vi "AlliGator Fit Linear Combinations of Exponentials.vi"(0 "Simulation Parameters":T1={"Decay Simulation Parameters"={"tau 1"=1e-09, "tau 2"=0.0, "a1"=1.0, "Baseline"=0.0}, "Fit Simulation Parameters"={"# Counts"=100, "# Simulations (N)"=100, "Decay Bin Size"=1.0000000000000002e-10, "# Bins"=200}, "Use Experimental IRF"=FALSE}, 5 "Decay Fit Options & Parameters":T5={"SYNC Period"=0.0, "Fit Options"={"Show Fit Residuals"=FALSE, "Fit Model"=enum."1-Exponential", "Residual Type"=enum."Standard", "Max Decay Percentile"=0.0, "Min Decay Percentile"=0.0, "Show Full Decay"=FALSE, "Weights"=enum."Unweighted", "Fitting Method"=enum."Least Square", "Compute Parameter Uncertainties"=FALSE, "Periodic Boundaries"=FALSE, "Model Calculation"=enum."Simulation", "Period"=0.0, "Termination Criteria"={"Max Iterations"=0, "Max Function Calls"=0, "Max Time"=0.0, "Function Tolerance"=0.0, "Parameter Tolerance"=0.0, "Gradient Tolerance"=0.0, "Min Lambda"=0.0, "Max Lambda"=0.0, "Initial Tick Count"=0}, "Offset Resolution"=0.0, "Use Local IRF"=FALSE, "Fitting Algorithm"=enum."Levenberg-Marquardt", "Show Confidence Interval "=TRUE, "Confidence Level"=95.0}, "Fit Parameter Constraints"=[], "MLE Baseline Offset"=0.0, "MLE Baseline Offset Type"=enum."Absolute"} {"Fit Options"."Confidence Level" min=0.0 max=100.0; "Fit Options"."Offset Resolution" min=0.0; "Fit Options"."Period" min=0.0; "Fit Options"."Min Decay Percentile" min=0.0 max=1.0; "Fit Options"."Max Decay Percentile" min=0.0 max=100.0; "Fit Parameter Constraints"."Max Value" format="%#.3g"; "Fit Parameter Constraints"."Min Value" format="%#.3g"}, 9 "Reference Decay":cluster{"t Array":dbl[], "IRF Array":dbl[]}, 11 "Error In":errorcluster, 12 "Show Decays, Fits & Residuals":bool) -> (1 "Output Plots":cluster{"t Array":dbl[], "I Array":dbl[]}[](array[cluster]), 2 "Output Plot Names":string[](array[string]), 3 "Plot Colors":u32[](array[colorbox]), 4 "Fit Results":T4[](array[typedef]), 6 "tau 1":dbl[](array[numeric]), 8 "tau 2":dbl[](array[numeric]), 10 "a 1":dbl[](array[numeric]), 14 "Message":string, 15 "Error Out":errorcluster)   [LabVIEW 2021, in "AlliGator Fit Method Benchmark.lvlib"]
doc: "Simulate a 1-Exp or 2-Exp decay and fits it with the selected model."
uses:
  AlliGator Fit Method Benchmark.lvlib
  Histograms/Histogram Bin Option.ctl
  Histograms/Histogram Window.lvlib
  Histograms/Histogram Bin Position.ctl
  Histograms/Linear Histogram Options.ctl
  Math/Math.lvlib
  GUI/GUI.lvlib
  Globals, Variables, Constants/AlliGator Abort.vi
  Globals, Variables, Constants/AlliGator Globals, Variables & Constants.lvlib
  Time/Time.lvlib
  Variant/Variant.lvlib
  Decay Analysis/Decay Fit/AlliGator Decay Fit.lvlib
  Graphs/XY Graph/XY Graph Refnum.ctl
  Graphs/XY Graph/XY Graph Add-Ons.lvlib
  <vilib>/Utility/miscctls.llb/LVPoint32TypeDef.ctl
  Graphs/XY Graph/XY Graph Selected Plot Info+Flag.ctl
  Fits/IRF(X)PSED/IRF(X)PSED Fit Results.ctl
  Fits/Fits.lvlib
  <vilib>/gmath/NI_Gmath.lvlib
  <vilib>/ErrorRing/Error Ring.xnode
  <vilib>/Utility/error.llb/Error Cluster From Error Code.vi
  Error/Error.lvlib
  <vilib>/gmath/statdist.llb/Exp Random.vi
  <vilib>/gmath/statdist.llb/Uniform (Discrete) Random.vi
  593261b4-01b2-4f61-a03e-748a91d26851.vi
  AlliGator FMB Global.vi
  AlliGator Fit Simulation Parameters.ctl
  AlliGator Decay Simulation Parameters.ctl
  Fits/IRF(X)PSED/Decay Fit Parameters In List.ctl
  Decay Analysis/Decay Fit/AlliGator Decay Fit Parameter Constraints 2.ctl
  Fits/Decay Convolution/Decay Model.ctl
  Fits/Residual Type.ctl
  Fits/Non-linear Fitting Method v2.ctl
  Fits/Fit Calculation Method.ctl
  Fits/Non-linear Fitting Algorithm.ctl
  Fits/IRF(X)PSED/MLE Baseline Offset Type.ctl
  AlliGator Simulation Parameters.ctl
  Fits/IRF(X)PSED/Fit Weights Type v2.ctl
  Fits/IRF(X)PSED/Decay Fit Options v4.ctl
  Decay Fit Parameter Map/AlliGator Decay Fit Options & Parameters v4.ctl
  Decay Fit Parameter Map/AlliGator Decay Fit Parameter Map.lvlib
panel:
  # "see the AlliGator License on the block diagram (Ctrl+E or Window:Show Block Diagram)"
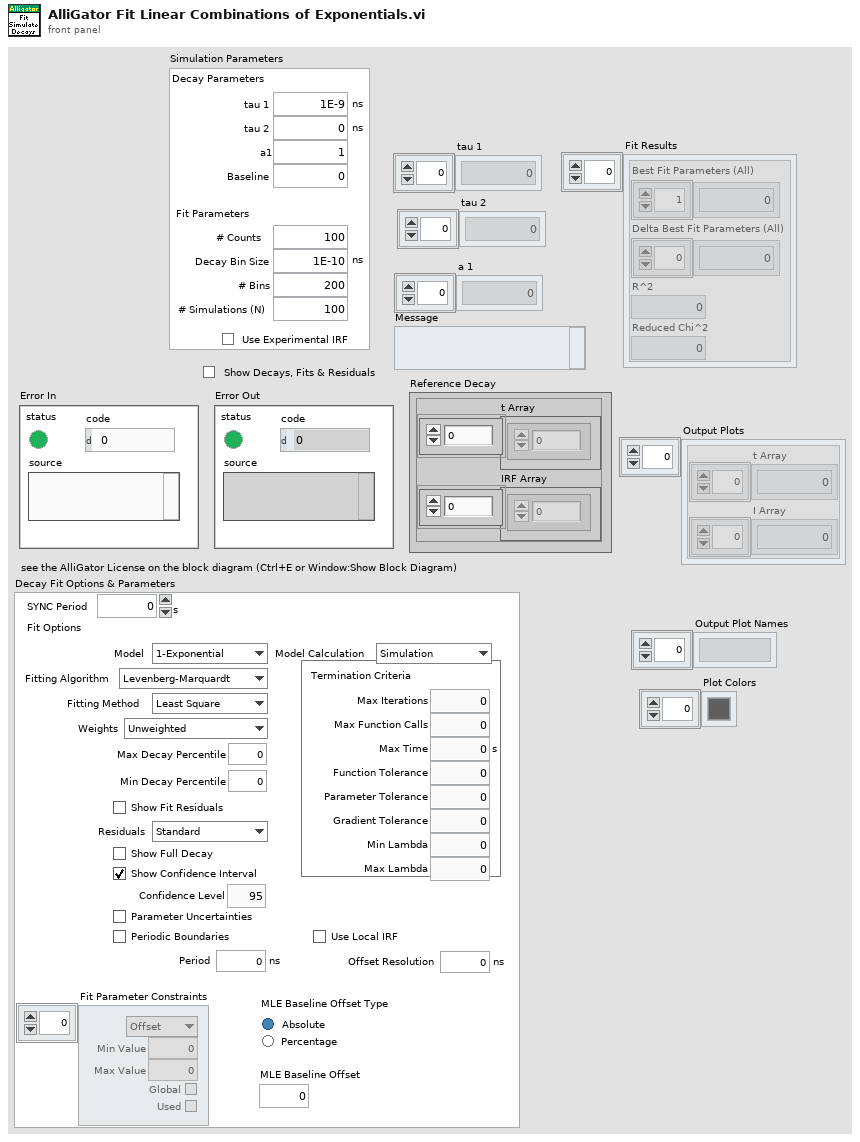
[diagram p1: front panel]
types:
  T1 = typedef "AlliGator Fit Method Benchmark.lvlib/AlliGator Simulation Parameters.ctl" = cluster{"Decay Simulation Parameters":T2, "Fit Simulation Parameters":T3, "Use Experimental IRF":bool}
  T2 = typedef "AlliGator Fit Method Benchmark.lvlib/AlliGator Decay Simulation Parameters.ctl" = cluster{"tau 1":dbl[unit], "tau 2":dbl[unit], "a1":dbl, "Baseline":dbl}
  T3 = typedef "AlliGator Fit Method Benchmark.lvlib/AlliGator Fit Simulation Parameters.ctl" = cluster{"# Counts":i32, "# Simulations (N)":i32, "Decay Bin Size":dbl[unit], "# Bins":i32}
  T4 = typedef "Fits.lvlib/IRF(X)PSED Fit Results.ctl" = cluster{"Best Fit Parameters (All)":dbl[], "Delta Best Fit Parameters (All)":dbl[], "R^2":dbl, "Reduced Chi^2":dbl}
  T5 = typedef "AlliGator Decay Fit Parameter Map.lvlib/AlliGator Decay Fit Options & Parameters v4.ctl" = cluster{"SYNC Period":dbl[unit], "Fit Options":T6, "Fit Parameter Constraints":T13[], "MLE Baseline Offset":dbl, "MLE Baseline Offset Type":T15}
  T6 = typedef "Fits.lvlib/Decay Fit Options v4.ctl" = cluster{"Show Fit Residuals":bool, "Fit Model":T7, "Residual Type":T8, "Max Decay Percentile":dbl, "Min Decay Percentile":dbl, "Show Full Decay":bool, "Weights":T9, "Fitting Method":T10, "Compute Parameter Uncertainties":bool, "Periodic Boundaries":bool, "Model Calculation":T11, "Period":dbl[unit], "Termination Criteria":cluster{"Max Iterations":i32, "Max Function Calls":i32, "Max Time":dbl[unit], "Function Tolerance":dbl, "Parameter Tolerance":dbl, "Gradient Tolerance":dbl, "Min Lambda":dbl, "Max Lambda":dbl, "Initial Tick Count":u32}, "Offset Resolution":dbl[unit], "Use Local IRF":bool, "Fitting Algorithm":T12, "Show Confidence Interval ":bool, "Confidence Level":dbl}
  T7 = typedef "Fits.lvlib/Decay Model.ctl" = enum16{"1-Exponential", "2-Exponentials"}
  T8 = typedef "Fits.lvlib/Residual Type.ctl" = enum16{"Standard", "Normalized", "Reduced"}
  T9 = typedef "Fits.lvlib/Fit Weights Type v2.ctl" = enum16{"Unweighted", "1/Variance (Neyman)", "1/Variance (Pearson)", "Best of All"}
  T10 = typedef "Fits.lvlib/Non-linear Fitting Method v2.ctl" = enum16{"Least Square", "Least Absolute Residual", "Bisquare", "MLE", "-", "Best of All"}
  T11 = typedef "Fits.lvlib/Fit Calculation Method.ctl" = enum16{"Simulation", "Convolution", "Integration"}
  T12 = typedef "Fits.lvlib/Non-linear Fitting Algorithm.ctl" = enum16{"Levenberg-Marquardt", "Trust-Region Dogleg"}
  T13 = typedef "AlliGator Decay Fit.lvlib/AlliGator Decay Fit Parameter Constraints 2.ctl" = cluster{"Fit Parameter":T14, "Min Value":dbl, "Max Value":dbl, "Global":bool, "Used":bool}
  T14 = typedef "Fits.lvlib/Decay Fit Parameters In List.ctl" = enum16{"Offset", "Baseline", "A_1", "tau_1", "A_2", "tau_2"}
  T15 = typedef "Fits.lvlib/MLE Baseline Offset Type.ctl" = enum32{"Absolute", "Percentage"}
  T16 = typedef "Histogram Window.lvlib/Linear Histogram Options.ctl" = cluster{"Bin Size":dbl, "Bin Number":i32, "Bin Option":T17, "Min Value":dbl, "Max Value":dbl, "Filter NaN & Infinite Values":bool, "Frequency Plot":bool, "Align Bins":bool, "Bin Location":T18, "Project Outside Values":bool, "Max Histogram Size":i32}
  T17 = typedef "Histogram Window.lvlib/Histogram Bin Option.ctl" = enum32{"Bin Number", "Bin Size"}
  T18 = typedef "Histogram Window.lvlib/Histogram Bin Position.ctl" = enum16{"Left", "Center", "Right"}
  T19 = typedef "XY Graph Add-Ons.lvlib/XY Graph Selected Plot Info+Flag.ctl" = cluster{"Multiplot XY Graph":T20, "Mouse Coordinates":T21, "Plot Index":i32, "Flag":bool}
  T20 = typedef "XY Graph Add-Ons.lvlib/XY Graph Refnum.ctl" = refnum<vi>
  T21 = typedef "LVPoint32TypeDef.ctl" = cluster{"Horizontal":i32, "Vertical":i32}
  T22 = typedef "XY Graph Add-Ons.lvlib/XY Graph Plot Data.ctl" = cluster{"X Array":dbl[], "Y Array":dbl[]}
  T23 = typedef "Fits.lvlib/Fit Plots.ctl" = cluster{"Fitted Decay":cluster{"t Array":dbl[], "Fitted Array":dbl[]}, "Residuals":cluster{"t Array":dbl[], "Residual Array":dbl[]}, "Upper CI Plot":cluster{"t Array":dbl[], "Residual Array":dbl[]}, "Lower CI Plot":cluster{"t Array":dbl[], "Residual Array":dbl[]}}
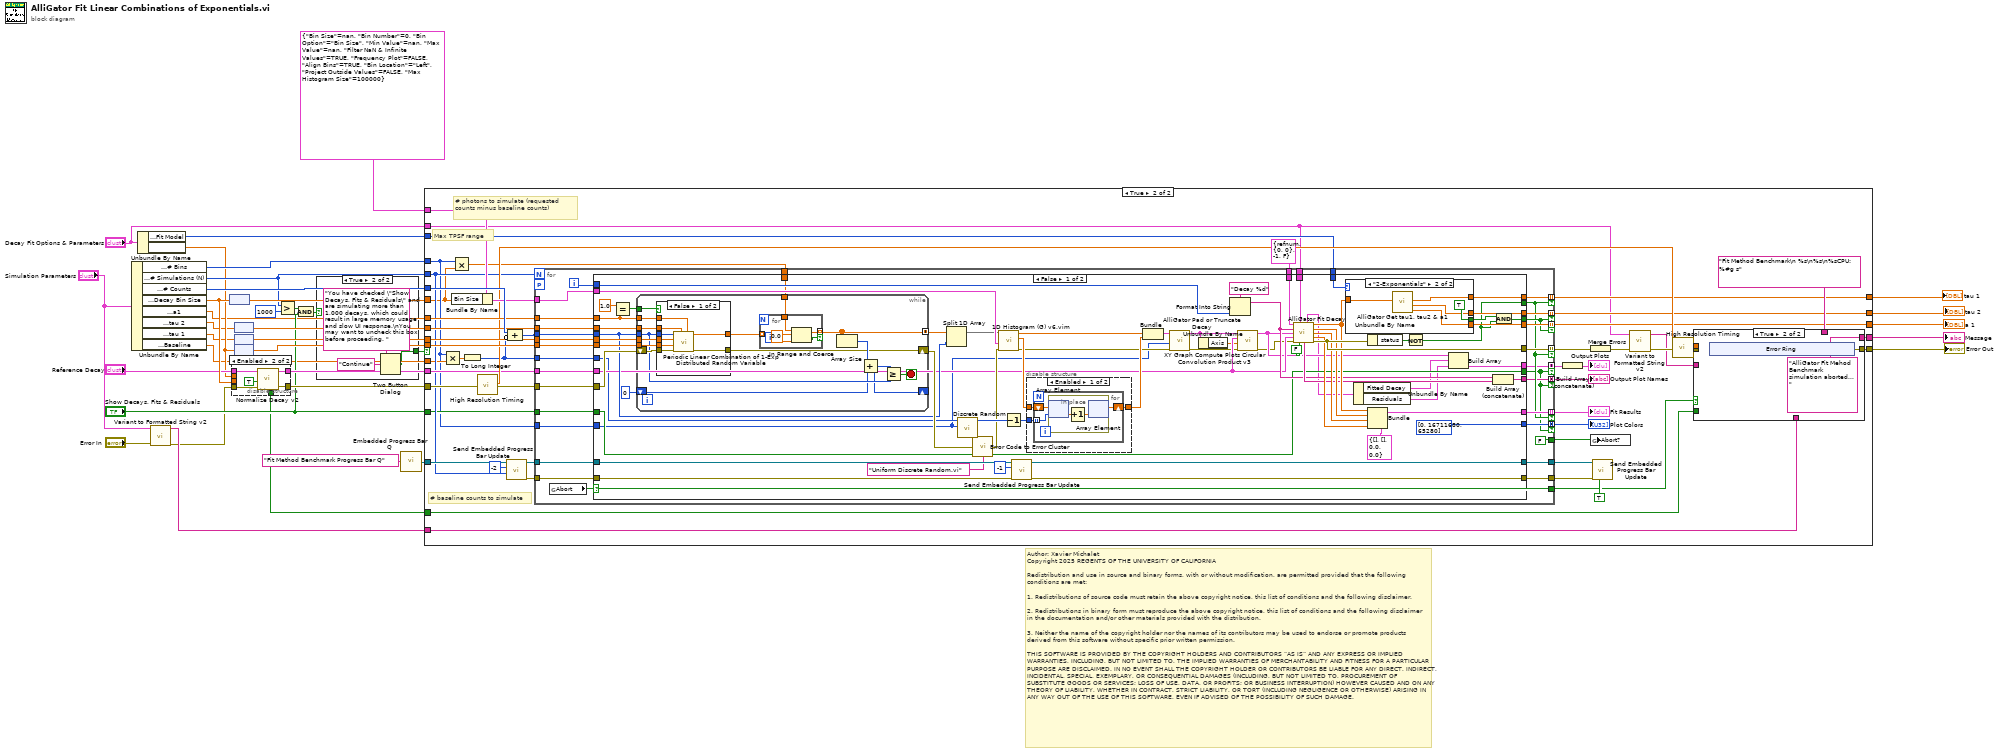
[diagram p0: block diagram]
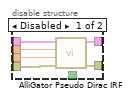
[diagram p2: hidden frame]
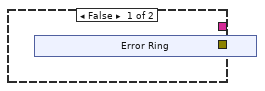
[diagram p3: hidden frame]
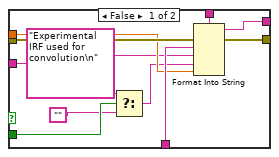
[diagram p4: hidden frame]
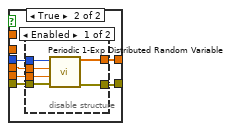
[diagram p5: hidden frame]
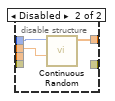
[diagram p6: hidden frame]
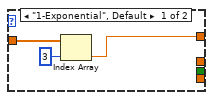
[diagram p8: hidden frame]
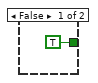
[diagram p10: hidden frame]
diagram:
  # "Author: Xavier Michalet\nCopyright 2025 REGENTS OF THE UNIVERSITY OF CALIFORNIA\n\nRedistribution and use in source and binary forms, with or without modification, are permitted provided that the following conditions are met:\n\n1. Redistributions of source code must retain the above copyright notice, this list of conditions and the following disclaimer.\n\n2. Redistributions in binary form must reproduce the above copyright notice, this list of conditions and the following disclaimer in the documentation and/or other materials provided with the distribution.\n\n3. Neither the name of the copyright holder nor the names of its contributors may be used to endorse or promote products derived from this software without specific prior written permission.\n\nTHIS SOFTWARE IS PROVIDED BY THE COPYRIGHT HOLDERS AND CONTRIBUTORS “AS IS” AND ANY EXPRESS OR IMPLIED WARRANTIES, INCLUDING, BUT NOT LIMITED TO, THE IMPLIED WARRANTIES OF MERCHANTABILITY AND FITNESS FOR A PARTICULAR PURPOSE ARE DISCLAIMED. IN NO EVENT SHALL THE COPYRIGHT HOLDER OR CONTRIBUTORS BE LIABLE FOR ANY DIRECT, INDIRECT, INCIDENTAL, SPECIAL, EXEMPLARY, OR CONSEQUENTIAL DAMAGES (INCLUDING, BUT NOT LIMITED TO, PROCUREMENT OF SUBSTITUTE GOODS OR SERVICES; LOSS OF USE, DATA, OR PROFITS; OR BUSINESS INTERRUPTION) HOWEVER CAUSED AND ON ANY THEORY OF LIABILITY, WHETHER IN CONTRACT, STRICT LIABILITY, OR TORT (INCLUDING NEGLIGENCE OR OTHERWISE) ARISING IN ANY WAY OUT OF THE USE OF THIS SOFTWARE, EVEN IF ADVISED OF THE POSSIBILITY OF SUCH DAMAGE."
  n1 = Unbundle By Name("Simulation Parameters") -> ("Fit Simulation Parameters.# Bins"=w9:i32, "Fit Simulation Parameters.# Simulations (N)"=w16:i32, "Fit Simulation Parameters.# Counts"=w36:i32, "Fit Simulation Parameters.Decay Bin Size"=w19:dbl[unit], "Decay Simulation Parameters.a1"=w5:dbl, "Decay Simulation Parameters.tau 2"=w4:dbl[unit], "Decay Simulation Parameters.tau 1"=w3:dbl[unit], "Decay Simulation Parameters.Baseline"=w2:dbl)
  n2 = Unbundle By Name("Decay Fit Options & Parameters") -> ("Fit Options.Fit Model"=w24:T7, "Fit Options.Period"=w7:dbl[unit])
  n3 = call "Variant to Formatted String v2.vi"("error in (no error)"="Error In", "Anything"="Simulation Parameters") -> ("error out"=w1:errorcluster, "String"=w25:string)  [unwired: 8 in]
  n4 = node(w19) -> (w31:dbl)
  n5 = disable-structure shown="Enabled" {
    disable-tunnel: [w42 w46] -> w20
    disable-tunnel: w19 -> [w41 _]
    disable-tunnel: "Reference Decay" -> [w40 w48]
    disable-tunnel: w1 -> [w39 w47]
    disable-tunnel: [w38 w45] -> w17
    disable-tunnel: w7 -> [w37 _]
    disable-tunnel: [_ w43] -> w8
    frame Disabled {
      n6 = call "AlliGator Pseudo Dirac IRF.vi"("Error In"=w39, "Decay Bin Size"=w41, "Period"=w37, "Reference Decay in"=w40) -> ("Error Out"=w38:errorcluster, "Reference Decay out"=w42:cluster{"t Array":dbl[], "IRF Array":dbl[]})  [unwired: 6 in]
    }
    frame Enabled {
      n7 = call "Normalize Decay v2.vi"("Error In"=w47, "Max = 1 (F)/Integral = 1 (T)"=TRUE, "Decay"=w48) -> ("Error Out"=w45:errorcluster, "Normalized Decay"=w46:cluster{"t Array":dbl[], "Y Array":dbl[]}, "Is Valid Plot?"=w43:bool)  [unwired: 4 in, 2 out]
    }
  }
  n8 = node(w4) -> (w32:dbl)
  n9 = node(w3) -> (w33:dbl)
  n10 = node(w7) -> (w35:dbl)
  n11 = Greater?(x=w16, y=1000) -> (0:w14:bool)
  n12 = And(x=w14, y="Show Decays, Fits & Residuals") -> (x .and. y?=w12:bool)
  n13 = case shown="True" w12 {
    tunnel: [TRUE ("T button?") w50] -> w11
    frame False {
    }
    frame True {
      n14 = Two Button Dialog(message="You have checked \"Show Decays, Fits & Residuals\" and are simulating more than 1,000 decays, which could result in large memory usage and slow UI response.\nYou may want to uncheck this box before proceeding. ", 2:"Continue" ("T button name (\"OK\")")) -> (T button?=w50:bool)  [unwired: 1 in]
    }
  }
  n15 = call "Embedded Progress Bar Q.vi"("Progress Bar Queue Name"="Fit Method Benchmark Progress Bar Q") -> ("Progress Bar Queue"=w29:refnum<queue>)  [unwired: 6 in]
  n16 = case shown="True" w11 {
    tunnel: w36 -> [_ w108]
    tunnel: w35 -> [_ w107]
    tunnel: T16 {"Bin Size"=nan, "Bin Number"=0, "Bin Option"=enum."Bin Size", "Min Value"=nan, "Max Value"=nan, "Filter NaN & Infinite Values"=TRUE, "Frequency Plot"=FALSE, "Align Bins"=TRUE, "Bin Location"=enum."Left", "Project Outside Values"=FALSE, "Max Histogram Size"=100000} ("Histogram Options") -> [_ w106]
    tunnel: w5 -> [_ w104]
    tunnel: w33 -> [_ w103]
    tunnel: w32 -> [_ w102]
    tunnel: w31 -> [_ w61]
    tunnel: w29 -> [_ w100]
    tunnel: [w53 w93] -> w28
    tunnel: [_ w92] -> w27
    tunnel: w25 -> [_ w91]
    tunnel: w24 -> [_ w82]
    tunnel: [_ w81] -> w23
    tunnel: [_ w80] -> w22
    tunnel: [_ w79] -> w21
    tunnel: "Decay Fit Options & Parameters" -> [_ w76]
    tunnel: w2 -> [_ w66]
    tunnel: w20 -> [_ w70]
    tunnel: w17 -> [_ w69]
    tunnel: w16 -> [_ w68]
    tunnel: "Show Decays, Fits & Residuals" -> [_ w67]
    tunnel: w9 -> [_ w62]
    tunnel: w8 -> [_ w59]
    frame False {
      n17 = xnode "Error Ring"() -> ("error out"=w53:errorcluster)
    }
    frame True {
      # "Max TPSF range"
      # "# photons to simulate (requested counts minus baseline counts)"
      # "# baseline counts to simulate"
      n18 = Multiply(x=w62, y=w66) -> (x*y=w65:dbl)
      n19 = Multiply(x=w62, y=w61) -> (x*y=w60:dbl)
      n20 = Bundle By Name(cluster=w106, "Bin Size"=w61) -> (w105:T16)
      n21 = To Long Integer(number=w65) -> (32bit integer=w63:i32)
      n22 = call "High Resolution Timing.vi"("Error In"=w69) -> ("elapsed (relative) seconds"=w87:dbl, "Error Out"=w89:errorcluster)  [unwired: 16 in, 1 out]
      n23 = call "Send Embedded Progress Bar Update.vi"("Max Iterations N"=w68, "Current Iteration i (i or -1: standard or || iteration; 0 or -2: first standard or || iteration)"=-2 ("Current Iteration i (-1: || iteration, -2: first || iteration)"), "Progress Bar Queue in"=w100) -> ("Error Out"=w97:errorcluster, "Progress Bar Queue out"=w99:refnum<queue>)  [unwired: 7 in]
      n24 = Compound Arithmetic op=ADD(w108, invert w63) -> (w64:i32)
      n25 = for {
        N: w68 -> [_]
        tunnel: w64 -> [w158]
        tunnel: w107 -> [w157]
        tunnel: w89 -> [w156]
        tunnel: w105 -> [w155]
        tunnel: w104 -> [w139]
        tunnel: w103 -> [w154]
        tunnel: w102 -> [w153]
        tunnel: w97 -> [w150]
        tunnel: [w149] -> w96
        tunnel: [FALSE ("Abort?")] -> w94
        tunnel: [w136] -> w85
        tunnel: w70 -> [w147]
        tunnel: w76 -> [w145]
        tunnel: [w138] -> w84 mode=indexing if=w134
        tunnel: T19 {"Multiplot XY Graph"=refnum, "Mouse Coordinates"={"Horizontal"=0, "Vertical"=0}, "Plot Index"=-1, "Flag"=FALSE} ("Selected Plot Info + Flag") -> [w144]
        tunnel: w82 -> [w143]
        tunnel: [w142] -> w81 mode=indexing if=w134
        tunnel: [w141] -> w80 mode=indexing if=w135
        tunnel: [w140] -> w79 mode=indexing if=w135
        tunnel: w99 -> [w152]
        tunnel: [w151] -> w98
        tunnel: [w137] -> w74 mode=indexing if=w134
        tunnel: [w133] -> w72 mode=concatenating if=w126
        tunnel: [w132] -> w73 mode=concatenating if=w126
        tunnel: w67 -> [w131]
        tunnel: [w130] -> w71 mode=concatenating if=w126
        tunnel: w63 -> [w129]
        tunnel: w62 -> [w128]
        tunnel: w60 -> [w127]
        workers-P: _ -> [_]
        i -> [w146]
        n26 = global read "AlliGator FMB Global.vi" "Abort"() -> (w136:bool)
        n27 = case shown="False" w136 {
          tunnel: w158 -> [w175 _]
          tunnel: w157 -> [w224 _]
          tunnel: w156 -> [w223 w287]
          tunnel: w155 -> [w222 _]
          tunnel: w154 -> [w221 _]
          tunnel: w153 -> [w220 _]
          tunnel: w152 -> [w218 w286]
          tunnel: [w217 w286] -> w151
          tunnel: w150 -> [w216 w285]
          tunnel: [w215 w285] -> w149
          tunnel: w147 -> [w173 _]
          tunnel: w146 -> [w214 _]
          tunnel: w145 -> [w212 _]
          tunnel: w144 -> [w210 _]
          tunnel: w143 -> [w209 _]
          tunnel: [w208 _] -> w142
          tunnel: [w207 _] -> w141
          tunnel: [w205 _] -> w140
          tunnel: w139 -> [w204 _]
          tunnel: [w201 w287] -> w138
          tunnel: [w199 _] -> w135
          tunnel: [w198 _] -> w134
          tunnel: [w192 _] -> w137
          tunnel: [w188 _] -> w133
          tunnel: [w189 _] -> w132
          tunnel: [w181 _] -> w126
          tunnel: w131 -> [w181 _]
          tunnel: [u32[] [0, 16711680, 65280] ("Plot Colors (Default)") _] -> w130
          tunnel: w129 -> [w168 _]
          tunnel: w128 -> [w165 _]
          tunnel: w127 -> [w182 _]
          frame False {
            n28 = Equal?(x=1.0, y=w204) -> (x = y?=w203:bool)
            n29 = while {
              tunnel: w224 -> [w239]
              tunnel: w221 -> [w237]
              tunnel: w220 -> [w236]
              tunnel: w204 -> [w235]
              tunnel: w203 -> [w234]
              tunnel: w182 -> [w232]
              tunnel: [w231] -> w180 mode=concatenating
              tunnel: w175 -> [w230]
              shift-right: [w225] -> w177
              shift-left: w223 -> [w238]
              shift-right: [w226] -> _
              shift-left: 0 -> [w227]
              stop <- w229 stop-if-true
              n30 = case shown="False" w234 {
                tunnel: w230 -> [w252 w256]
                tunnel: w239 -> [w251 w254]
                tunnel: w238 -> [w250 w258]
                tunnel: [w249 w253] -> w233
                tunnel: [w248 w257] -> w225
                tunnel: w237 -> [w247 w255]
                tunnel: w236 -> [w246 _]
                tunnel: w235 -> [w245 _]
                frame False {
                  n31 = call "Periodic Linear Combination of 1-Exp Distributed Random Variable.vi"("a 1 (in [0, 1])"=w245, "tau 2"=w246, "Error In"=w250, "T"=w251, "tau 1"=w247, "# Elements"=w252) -> ("Error Out"=w248:errorcluster, "t Array"=w249:dbl[])  [unwired: 4 in]
                }
                frame True {
                  n32 = disable-structure shown="Enabled" {
                    disable-tunnel: w258 -> [w264 _]
                    disable-tunnel: [w263 _] -> w257
                    disable-tunnel: w256 -> [w262 w267]
                    disable-tunnel: w255 -> [w261 w266]
                    disable-tunnel: w254 -> [w260 _]
                    disable-tunnel: [w259 w265] -> w253
                    frame Enabled {
                      n33 = call "Periodic 1-Exp Distributed Random Variable.vi"("Error In"=w264, "T"=w260, "tau"=w261, "# Elements"=w262) -> ("Error Out"=w263:errorcluster, "t Array"=w259:dbl[])  [unwired: 6 in]
                    }
                    frame Disabled {
                      n34 = call-poly <vilib>:"Continuous Random.vi"("b"=w266, "samples"=w267) -> ("exp random data"=w265:dbl[])  [unwired: 8 in, 1 out]
                    }
                  }
                }
              }
              n35 = for {
                tunnel: w233 -> [w243] mode=indexing
                tunnel: w232 -> [w244]
                tunnel: [w241] -> w231 mode=indexing if=w240
                n36 = In Range and Coerce(upper limit=w244, x=w243, lower limit=0.0 ("x")) -> (coerced(x)=w241:dbl, In Range?=w240:bool)
              }
              n37 = Array Size(array=w231) -> (size(s)=w228:i32)
              n38 = Add(x=w228, y=w227) -> (x+y=w226:i32)
              n39 = Greater Or Equal?(x=w226, y=w230) -> (x >= y?=w229:bool)
            }
            n40 = Split 1D Array(array=w180, index=w175) -> (first subarray=w174:dbl[])  [unwired: 1 out]
            n41 = call-poly <vilib>:"Discrete Random.vi"("n"=w165, "samples"=w168) -> ("error"=w178:i32, "uniform (discrete) random data"=w186:i32[])  [unwired: 8 in]
            n42 = call "Error Code to Error Cluster.vi"("Error Code"=w178, "Error Source"="Uniform Discrete Random.vi", "Error In"=w177) -> ("Error Out"=w176:errorcluster)  [unwired: 12 in]
            n43 = call "1D Histogram (G) v6.vim"("Error In"=w176, "Histogram Options"=w222, "Array"=w174) -> ("Error Out"=w167:errorcluster, "Histogram"=w184:dbl[], "Axis"=w169:dbl[])  [unwired: 2 in, 4 out]
            n44 = Decrement(x=w186) -> (x-1=w185:i32[])
            n45 = call "Send Embedded Progress Bar Update.vi"("Error In"=w216, "Current Iteration i (i or -1: standard or || iteration; 0 or -2: first standard or || iteration)"=-1 ("Current Iteration i (i or -1: standard or || iteration; 0 or -2: first standard or || iteration)"), "Progress Bar Queue in"=w218) -> ("Error Out"=w215:errorcluster, "Progress Bar Queue out"=w217:refnum<queue>)  [unwired: 7 in]
            n46 = disable-structure shown="Enabled" {
              disable-tunnel: w185 -> [w270 _]
              disable-tunnel: w184 -> [w269 w276]
              disable-tunnel: [w268 w276] -> w183
              frame Enabled {
                n47 = for {
                  tunnel: w270 -> [w271] mode=indexing
                  shift-right: [w272] -> w268
                  shift-left: w269 -> [w273]
                  n48 = in-place {
                    n49 = in-place-array #1(w273, w271) -> (w275:dbl)
                    n50 = Increment(x=w275) -> (x+1=w274:dbl)
                    n51 = in-place-array #1(w274) -> (w272:dbl[])  [unwired: 1 out]
                  }
                }
              }
              frame Disabled {
              }
            }
            n52 = Bundle("Axis"=w169, "Histogram"=w183) -> (w170:cluster{"Axis":dbl[], "Histogram":dbl[]})  [unwired: 1 in]
            n53 = call "AlliGator Pad or Truncate Decay.vi"("Error In"=w167, "# Requested Points"=w165, "Plot in"=w170) -> ("Error Out"=w166:errorcluster, "Plot out"=w164:cluster{"Axis":dbl[], "Histogram":dbl[]})  [unwired: 7 in]
            n54 = Unbundle By Name(w164) -> ("Axis"=w163:dbl[])
            n55 = Format Into String(format string="Decay %d", w214) -> (resulting string=w187:string)  [unwired: 2 in, 1 out]
            n56 = call "XY Graph Compute Plots Circular Convolution Product v3.vi"("Error In"=w166, "Support Axis (kernel's)"=w163, "Plot 2 (kernel)"=w173, "Plot 1 (function)"=w164) -> ("Error Out"=w171:errorcluster, "Convolution Product"=w172:T22)  [unwired: 5 in, 1 out]
            n57 = call "AlliGator Fit Decay.vi"("Selected Plot Info + Flag"=w210, "Decay Fit Options & Parameters"=w212, "Current Decay Name"=w187, "Current Decay"=w172, "Reference Decay"=w173, "error in (no error)"=w171, "Use Legacy Fitting Approach"=FALSE) -> ("Fit Plots"=w161:T23, "Best Fit Parameters (All)"=w197:dbl[], "Delta Best Fit Parameters (All)"=w196:dbl[], "R^2"=w195:dbl, "Reduced Chi^2"=w194:dbl, "Output Plot Names"=w191:string[], "Error Out"=w201:errorcluster)  [unwired: 2 out]
            n58 = case shown="\"2-Exponentials\"" w209 {
              tunnel: w197 -> [w279 w283]
              tunnel: [w277 w282] -> w208
              tunnel: [_ w281] -> w207
              tunnel: [_ TRUE] -> w206
              tunnel: [_ w280] -> w205
              frame "1-Exponential", Default {
                n59 = Index Array(array=w279, index=3) -> (element=w277:dbl)
              }
              frame "2-Exponentials" {
                n60 = call "AlliGator Get tau1, tau2 & a1.vi"("Best Fit Parameters"=w283) -> ("a 1"=w280:dbl, "tau 2"=w281:dbl, "tau 1"=w282:dbl)  [unwired: 8 in]
              }
            }
            n61 = Unbundle By Name(w161) -> ("Fitted Decay"=w160:cluster{"t Array":dbl[], "Fitted Array":dbl[]}, "Residuals"=w159:cluster{"t Array":dbl[], "Residual Array":dbl[]})
            n62 = Unbundle By Name(w201) -> ("status"=w200:bool)
            n63 = Bundle(cluster=T4 {"Best Fit Parameters (All)"=[], "Delta Best Fit Parameters (All)"=[], "R^2"=0.0, "Reduced Chi^2"=0.0} ("output cluster"), "Best Fit Parameters (All)"=w197, "Delta Best Fit Parameters (All)"=w196, "R^2"=w195, "Reduced Chi^2"=w194) -> (w192:T4)
            n64 = Not(x=w200) -> (.not. x?=w198:bool)
            n65 = Build Array(w172, w160, w159) -> (w189:T22[])
            n66 = Build Array (concatenate)(w187, w191) -> (w188:string[])
            n67 = And(x=w206, y=w198) -> (x .and. y?=w199:bool)
          }
          frame True {
          }
        }
      }
      "Fit Results" <- w74
      "Output Plot Names" <- w72
      "Plot Colors" <- w71
      n68 = Build Array (concatenate)(w73) -> (→"Output Plots":T22[])
      n69 = Merge Errors(w84) -> (w78:errorcluster)
      n70 = global write "AlliGator Abort.vi" "Abort?"(w94) -> ()
      n71 = call "Send Embedded Progress Bar Update.vi"("Stop Progress Bar (F)"=TRUE, "Error In"=w96, "Progress Bar Queue in"=w98) -> ()  [unwired: 7 in, 2 out]
      n72 = call "Variant to Formatted String v2.vi"("error in (no error)"=w78, "Anything"=w76) -> ("error out"=w77:errorcluster, "String"=w75:string)  [unwired: 8 in]
      n73 = call "High Resolution Timing.vi"("relative seconds (NaN)"=w87, "Error In"=w77) -> ("elapsed (relative) seconds"=w86:dbl, "Error Out"=w88:errorcluster)  [unwired: 15 in, 1 out]
      n74 = case shown="True" w85 {
        tunnel: [w119 w120] -> w93
        tunnel: [w118 "AlliGator Fit Mehod Benchmark simulation aborted..."] -> w92
        tunnel: w91 -> [w117 _]
        tunnel: "Fit Method Benchmark\n %s\n%s\n%sCPU: %#g s" ("format string") -> [w116 _]
        tunnel: w88 -> [w115 _]
        tunnel: w86 -> [w114 _]
        tunnel: w75 -> [w113 _]
        tunnel: w59 -> [w112 _]
        frame False {
          n75 = Select(t="Experimental IRF used for convolution\n", s=w112, f="") -> (s? t:f=w111:string)
          n76 = Format Into String(format string=w116, error in=w115, w117, w113, w111, w114) -> (resulting string=w118:string, error out=w119:errorcluster)  [unwired: 1 in]
        }
        frame True {
          n77 = xnode "Error Ring"() -> ("error out"=w120:errorcluster)
        }
      }
    }
  }
  "Error Out" <- w28
  "a 1" <- w21
  "tau 1" <- w23
  "tau 2" <- w22
  "Message" <- w27
